vi "U3 easy Stream Example.vi"() -> ()   [LabVIEW 2021]
panel:
  out "Data":dbl[][](array[numeric]) format="%.3f"
  out "Waveform Graph":dbl[][](graph)
  in  "Scan List (+)":u8[](array[numeric])=[0, 1, 2, 3]
  out "# of iterations":i32
  in  "Scan Rate (Hz)":dbl=1000.0 format="%.3f"
  in  "stop":bool
  out "Error Message":string
  # "This example streams from the first found USB U3.  Streaming\nrequires U3 hardware revision 1.21+."
  # "The + scan list is the positive\nchannels.  For each element in\nthe + list, there must also be\nan element in the - list, which is\nthe negative channels.  For\nsingle-ended channels, put in\n31 for the negative channel.\n\nTo remove an element, right-click\non it, select Data Operations =>\nRemove Element.\n\nTo empty an array, right-click\nnear the edge, select Data\nOperations => Empty Array.\n\nOther useful operations:  From the\nOperate menu are \"Make Current\nValues Default\" and \"Reinitialize\nTo Default\"."
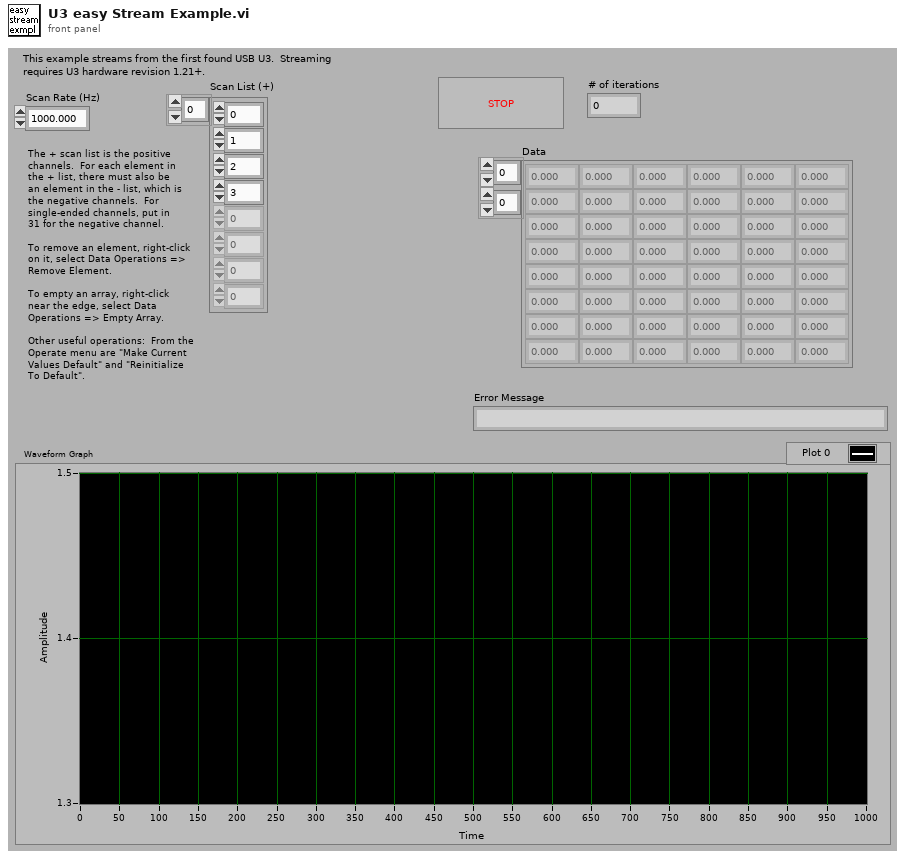
[diagram p1: front panel]
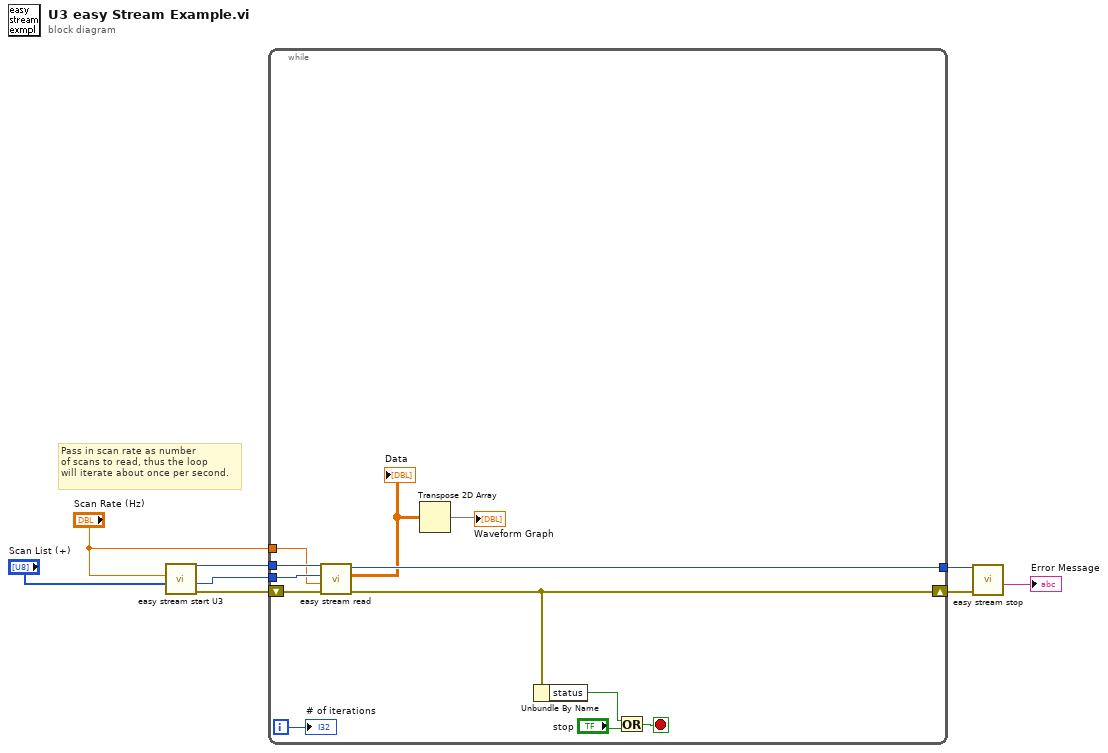
[diagram p0: block diagram]
diagram:
  # "Pass in scan rate as number\nof scans to read, thus the loop\nwill iterate about once per second."
  n1 = call "easy stream start U3.vi"("Scan List (+)"="Scan List (+)", "Scan Rate (Hz)"="Scan Rate (Hz)") -> ("error out"=w8:errorcluster, "# Channels"=w6:i32, "Handle Out"=w5:i32)  [unwired: 6 in, 1 out]
  n2 = while {
    tunnel: "Scan Rate (Hz)" -> [w9]
    tunnel: [w12] -> w3
    tunnel: w5 -> [w13]
    tunnel: w6 -> [w14]
    shift-left: w8 -> [w15]
    shift-right: [w10] -> w4
    i -> [w17]
    stop <- w18 stop-if-true
    n3 = call "easy stream read.vi"("error in"=w15, "Scans To Read"=w9, "# Channels In Stream"=w14, "Handle In"=w13) -> ("error out"=w10:errorcluster, "Data"=w11:dbl[][], "Handle Out"=w12:i32)  [unwired: 4 in, 1 out]
    "Data" <- w11
    n4 = Transpose 2D Array(2D array=w11) -> (transposed array=→"Waveform Graph":dbl[][])
    n5 = Unbundle By Name(w10) -> ("status"=w19:bool)
    n6 = Or(x=w19, y="stop") -> (x .or. y?=w18:bool)
    "# of iterations" <- w17
  }
  n7 = call "easy stream stop.vi"("error in"=w4, "Handle In"=w3) -> ("Error Message"=→"Error Message":string)  [unwired: 7 in, 2 out]
